vi "close_all_data_queue.vi"(8 "error in (no error)":errorcluster, 11 "data_queue":cluster{"AnalogReadData":refnum<queue>}) -> (0 "error out":errorcluster)   [LabVIEW 2017]
doc: "Close all data queues"
uses:
  measurement_result/MeasurementResult.lvclass
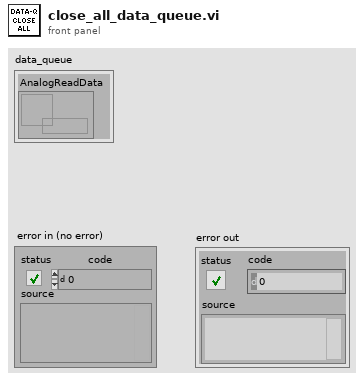
[diagram p1: front panel]
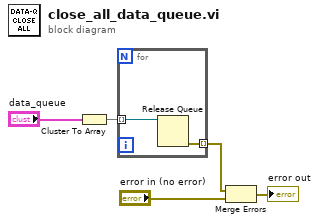
[diagram p0: block diagram]
diagram:
  n1 = Cluster To Array(cluster="data_queue") -> (array=w4:refnum<queue>[])
  n2 = for {
    tunnel: w4 -> [w7] mode=indexing
    tunnel: [w6] -> w3 mode=indexing
    n3 = Release Queue(queue=w7) -> (error out=w6:errorcluster)  [unwired: 2 in, 2 out]
  }
  n4 = Merge Errors(w3, "error in (no error)") -> (→"error out":errorcluster)
